vi "Configure Measurement (Intermod).vi"(0 "VISA resource name":refnum<visa-resource-name>, 5 "Intermod Span (15 MHz)":dbl=15000000.0 format="%#.6g", 7 "Enable Auto Max Mixer Level (T: Enable)":bool=TRUE, 9 "Max Mixer Level (-30 dBm)":dbl=-30.0 format="%#.6g", 11 "error in (no error)":errorcluster) -> (4 "VISA resource name out":refnum<visa-resource-name>, 15 "error out":errorcluster)   [LabVIEW 2014, in "Agilent ESA PSA Series.lvlib"]
doc: "Sets up the third order intercept points measurement."
uses:
  Agilent ESA PSA Series.lvlib
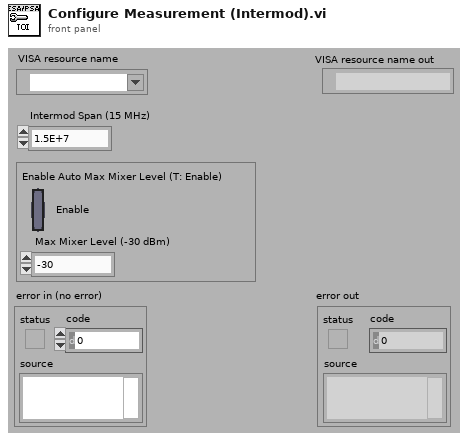
[diagram p1: front panel]
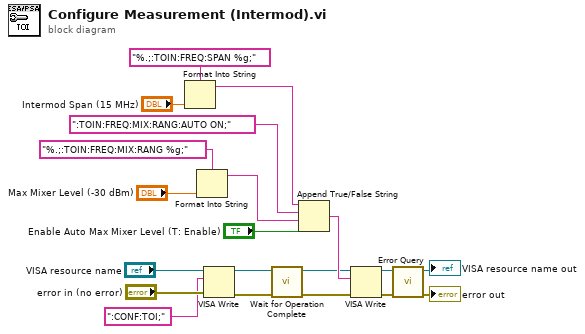
[diagram p0: block diagram]
diagram:
  n1 = Format Into String(format string="%.;:TOIN:FREQ:SPAN %g;", "Intermod Span (15 MHz)") -> (resulting string=w13:string)  [unwired: 2 in, 1 out]
  n2 = Format Into String(format string="%.;:TOIN:FREQ:MIX:RANG %g;", "Max Mixer Level (-30 dBm)") -> (resulting string=w15:string)  [unwired: 2 in, 1 out]
  n3 = VISA Write(VISA resource name="VISA resource name", write buffer=":CONF:TOI;" ("initial string"), error in (no error)="error in (no error)") -> (VISA resource name out=w5:refnum<visa-resource-name>, error out=w4:errorcluster)  [unwired: 1 out]
  n4 = call "Wait for Operation Complete.vi"("error in (no error)"=w4, "VISA resource name"=w5) -> ("error out"=w2:errorcluster, "VISA resource name out"=w3:refnum<visa-resource-name>)  [unwired: 8 in]
  n5 = Append True/False String(1:"Enable Auto Max Mixer Level (T: Enable)", 2:w15, 3:":TOIN:FREQ:MIX:RANG:AUTO ON;" ("initial string"), 4:w13) -> (0:w10:string)
  n6 = VISA Write(VISA resource name=w3, write buffer=w10, error in (no error)=w2) -> (VISA resource name out=w9:refnum<visa-resource-name>, error out=w8:errorcluster)  [unwired: 1 out]
  n7 = call "Error Query.vi"("error in (no error)"=w8, "VISA resource name"=w9) -> ("error out"=→"error out":errorcluster, "VISA resource name out"=→"VISA resource name out":refnum<visa-resource-name>)  [unwired: 6 in, 2 out]
